vi "set_alignment_wavelength.vi"(8 "error in (no error)":errorcluster, 10 "wavelength in":dbl[unit], 11 "LightSourceAN191011Chameleon in":refnum<class "LightSourceAN191011Chameleon.lvclass">) -> (0 "error out":errorcluster, 3 "LightSourceAN191011Chameleon out":refnum<class "LightSourceAN191011Chameleon.lvclass">)   [LabVIEW 2010, in "LightSourceAN191011Chameleon.lvclass"]
uses:
  LightSourceAN191011Chameleon.lvclass
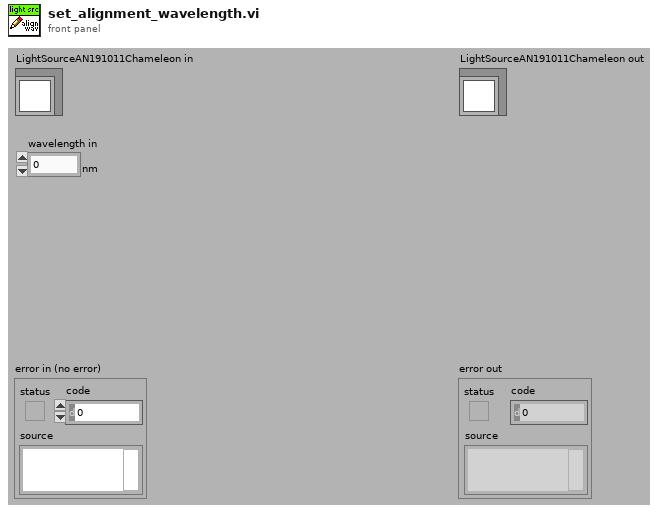
[diagram p1: front panel]
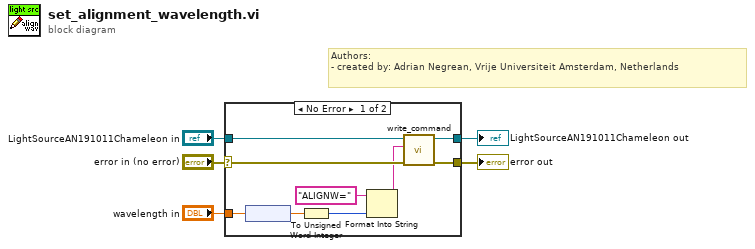
[diagram p0: block diagram]
diagram:
  # "Authors: \n- created by: Adrian Negrean, Vrije Universiteit Amsterdam, Netherlands"
  n1 = case shown="No Error" "error in (no error)" {
    selector: "error in (no error)" -> [w14 w16]
    tunnel: [w13 w16] -> w4
    tunnel: [w11 w15] -> w2
    tunnel: "LightSourceAN191011Chameleon in" -> [w12 w15]
    tunnel: "wavelength in" -> [w10 _]
    frame No Error {
      n2 = node(w10) -> (w9:dbl)
      n3 = To Unsigned Word Integer(number=w9) -> (unsigned 16bit integer=w8:u16)
      n4 = Format Into String(initial string="ALIGNW=" ("string"), w8) -> (resulting string=w6:string)  [unwired: 2 in, 1 out]
      n5 = call-dynamic "write_command.vi"("error in (no error)"=w14, "string to write"=w6, "LightSourceAN191011Chameleon in"=w12) -> ("error out"=w13:errorcluster, "LightSourceAN191011Chameleon out"=w11:refnum<class "LightSourceAN191011Chameleon.lvclass">)  [unwired: 6 in, 1 out]
    }
    frame Error {
    }
  }
  "error out" <- w4
  "LightSourceAN191011Chameleon out" <- w2
